vi "SetSerialTermChar.vi"(8 "error IO":errorcluster {"code" format="%.0x"}, 9 "termination char\n(0xA = '\\n' = LF)":u8=10 format="%.0x", 11 "VISA resource name":refnum<visa-resource-name>) -> (0 "error IO 2":errorcluster {"code" format="%.0x"})   [LabVIEW 2015, in "Agilent 546XX Series.lvlib"]
uses:
  Agilent 546XX Series.lvlib
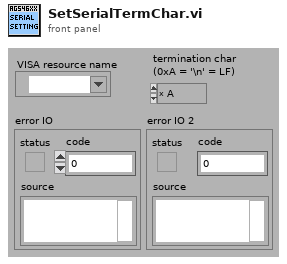
[diagram p1: front panel]
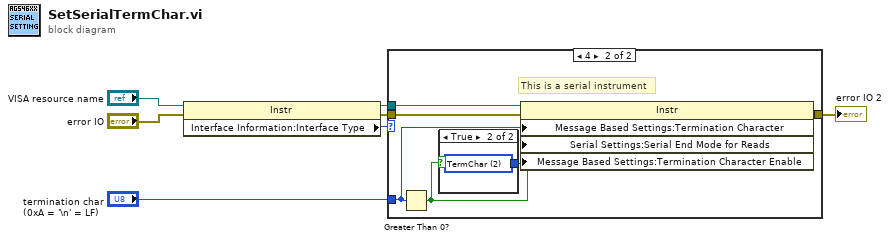
[diagram p0: block diagram]
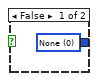
[diagram p3: hidden frame]
diagram:
  n1 = property class="Instr"(reference="VISA resource name", error in="error IO") -> (reference out=w5:refnum<visa-resource-name>, error out=w2:errorcluster, "Interface Information:Interface Type"=w4:u16)
  n2 = case shown="4" w4 {
    tunnel: w5 -> [_ w14]
    tunnel: "termination char\n(0xA = '\\n' = LF)" -> [_ w13]
    tunnel: w2 -> [w8 w12]
    tunnel: [w8 w11] -> w1
    frame 0, Default {
      # "This is a non-serial instrument"
    }
    frame 4 {
      # "This is a serial instrument"
      n3 = Greater Than 0?(x=w13) -> (x > 0?=w10:bool)
      n4 = case shown="True" w10 {
        tunnel: [w15 w16] -> w9
        frame False {
          w15 = u16 0 items=["None", "LastBit", "TermChar"] ("Serial Settings:Serial End Mode for Reads")
        }
        frame True {
          w16 = u16 2 items=["None", "LastBit", "TermChar"] ("Serial Settings:Serial End Mode for Reads")
        }
      }
      n5 = property class="Instr"(reference=w14, error in=w12, "Message Based Settings:Termination Character"=w13, "Serial Settings:Serial End Mode for Reads"=w9, "Message Based Settings:Termination Character Enable"=w10) -> (error out=w11:errorcluster)  [unwired: 1 in]
    }
  }
  "error IO 2" <- w1
